vi "GetAuxGlobals.vi"() -> (1 "ShooterSpeedDemand":dbl, 2 "ShooterRPM":dbl)   [LabVIEW 2020]
uses:
  AuxGlobals.vi
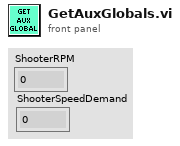
[diagram p1: front panel]
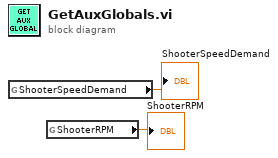
[diagram p0: block diagram]
diagram:
  n1 = global read "AuxGlobals.vi" "ShooterSpeedDemand"() -> (→"ShooterSpeedDemand":dbl)
  n2 = global read "AuxGlobals.vi" "ShooterRPM"() -> (→"ShooterRPM":dbl)
